vi "PH_AxisGUI_NF.constructor.vi"(0 "name":string, 2 "data in":string, 5 "error in(no error)":errorcluster) -> (14 "i ref out":refnum<vi>, 16 "data out":string, 19 "error out":errorcluster)   [LabVIEW 2014, in "PH_AxisGUI_NF.lvlib"]
doc: "This class is forseen to control up to three New Focus motors (class: NF87xx).\n\nThis class is part of the PHELIX user layer.\n\nauthor: Stefan Götte, GSI\n\nLicense Agreement for this software:\n\nCopyright (C)\nGesellschaft für Schwerionenforschung, GSI\nPlanckstr. 1\n64291 Darmstadt\nGermany\n\nContact: D.Beck@gsi.de \n\nThis program is free software; you can redistribute it and/or modify it under the terms of the \nGNU General Public License as published by the Free Software Foundation; either version 2 of \nthe license, or (at your option) any later version.\n\nThis program is distributed in the hope that it will be useful, but WITHOUT ANY WARRANTY; \nwithout even the implied warranty of MERCHANTABILITY or FITNESS FOR A PARTICULAR PURPOSE. See the GNU General License for more details (http://www.gnu.org).\n\nGesellschaft für Schwerionenforschung, GSI\nPlanckstr. 1, 64291 Darmstadt, Germany\nFor all questions and ideas contact: M.Richter@gsi.de, H.Brand@gsi.de or D.Beck@gsi.de.\nLast update: 16-JUN-2004"
uses:
  PH_AxisGUI_NF.lvlib
  CS_Core/CSObj/CSObj.lvlib
  PH_Basics/PH_Class/PH_Class.lvlib
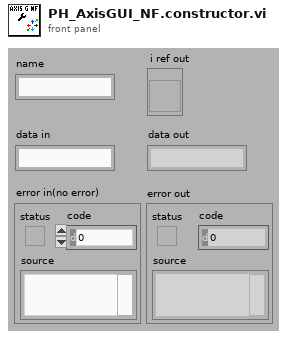
[diagram p1: front panel]
types:
  T1 = enum16{"SetAttribute", "GetAttribute", "CreateAttribute", "DestroyAttribute", "DestroyAllAtributes"}
  T2 = typedef "PH_AxisGUI_NF.lvlib/PH_AxisGUI_NF.i attribute.ctl" = cluster{"GUI Refs":cluster{"Delete":refnum<vi>, "Slide 0":refnum<vi>, "Slide 1":refnum<vi>, "Slide 2":refnum<vi>, "Instance Status":refnum<vi>, "Position":refnum<vi>, "Reset":refnum<vi>, "Goal":refnum<vi>, "Go":refnum<vi>}, "Instance":string, "Name Axis 0":string, "Name Axis 1":string, "Name Axis 2":string, "System":string, "Driver Type":T3, "Offset":i32, "Goal":i32}
  T3 = typedef "NF87XX.lvlib/NF87XX.driver Type.ctl" = enum16{"not defined", "3-ch open loop drv", "1-ch closed loop drv"}
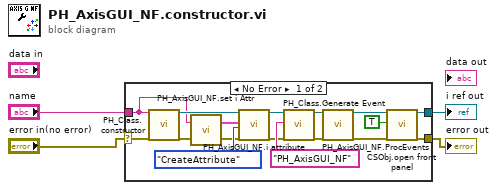
[diagram p0: block diagram]
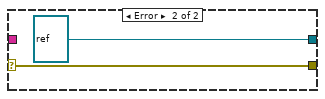
[diagram p2: hidden frame]
diagram:
  n1 = case shown="No Error" "error in(no error)" {
    selector: "error in(no error)" -> [w17 w23]
    tunnel: "name" -> [w5 _]
    tunnel: [w19 refnum<vi> refnum ("i ref out")] -> w3
    tunnel: [w18 w23] -> w2
    frame No Error {
      n2 = call "PH_Class.constructor.vi"("name"=w5, "error in"=w17) -> ("i ref out"=w6:refnum<vi>, "error out"=w10:errorcluster)  [unwired: 15 in, 1 out]
      n3 = call "PH_AxisGUI_NF.set i Attr.vi"("error in (no error)"=w10, "DB Entry to read"=w5) -> ("error out"=w9:errorcluster, "i Attributes"=w8:T2)
      n4 = call "PH_AxisGUI_NF.i attribute.vi"("VI Refnum"=w6, "CLASS.i attribute"=w8, "Action"=T1."CreateAttribute", "error in (no error)"=w9) -> ("VI Refnum out"=w11:refnum<vi>, "error out"=w7:errorcluster)  [unwired: 13 in, 1 out]
      n5 = call "PH_Class.Generate Event.vi"("i ref in"=w11, "Class"="PH_AxisGUI_NF", "error in (no error)"=w7) -> ("i ref out"=w16:refnum<vi>, "error out"=w15:errorcluster)  [unwired: 15 in]
      n6 = call "PH_AxisGUI_NF.ProcEvents.vi"("i ref in"=w16, "error in"=w15) -> ("i ref out"=w13:refnum<vi>, "error out"=w12:errorcluster)  [unwired: 16 in]
      n7 = call "CSObj.open front panel.vi"("i ref in"=w13, "frontPanelOpen"=TRUE ("front panel open"), "error in (no error)"=w12) -> ("i ref out"=w19:refnum<vi>, "error out"=w18:errorcluster)  [unwired: 15 in]
    }
    frame Error {
    }
  }
  "i ref out" <- w3
  "error out" <- w2
